vi "LDF Get Frame Name.vi"(9 "pFrameName":string, 10 "index":i32, 11 "LDFHandle":u64) -> (1 "pFrameName out":string, 3 "function return":i32)   [LabVIEW 2010, in "ldf_parser.lvlib"]
doc: "int WINAPI LDF_GetFrameName(long long LDFHandle, int index, char* pFrameName);"
uses:
  ldf_parser.lvlib
  USB2XXX/trunk/USB2XXX/USB2XXX/vs2019/Release/USB2XXX.dll
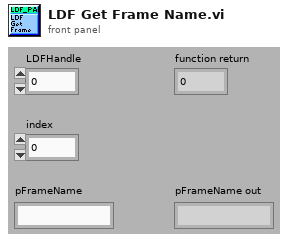
[diagram p1: front panel]
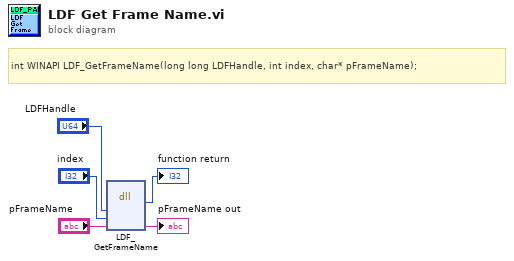
[diagram p0: block diagram]
diagram:
  # "int WINAPI LDF_GetFrameName(long long LDFHandle, int index, char* pFrameName);"
  n1 = dll-call lib="E:/Projects/USB2XXX/trunk/USB2XXX/USB2XXX/vs2019/Release/USB2XXX.*" fn="LDF_GetFrameName"("LDFHandle"="LDFHandle", "index"="index", "pFrameName"="pFrameName") -> (→"function return":i32, "pFrameName"=→"pFrameName out":string)  [unwired: 5 in, 2 out]
